vi "LabvolutionSubmoduleCheck_AddSubmoduleDialog.vi"(8 "error in (no error)":errorcluster, 11 "Project Dir":path) -> (0 "error out":errorcluster)   [LabVIEW 2018]
panel:
  in  "Select submodule parent folder":string(combo)
  in  "Cancel":bool
  in  "Add submodule":bool
  in  "Repository URL":string
  # "C:\\Users\\GregPayne\\Documents\\grp\\tmp\\submodule-demo"
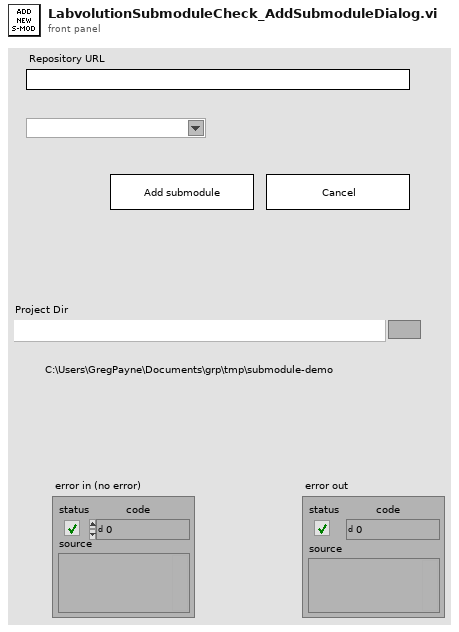
[diagram p1: front panel]
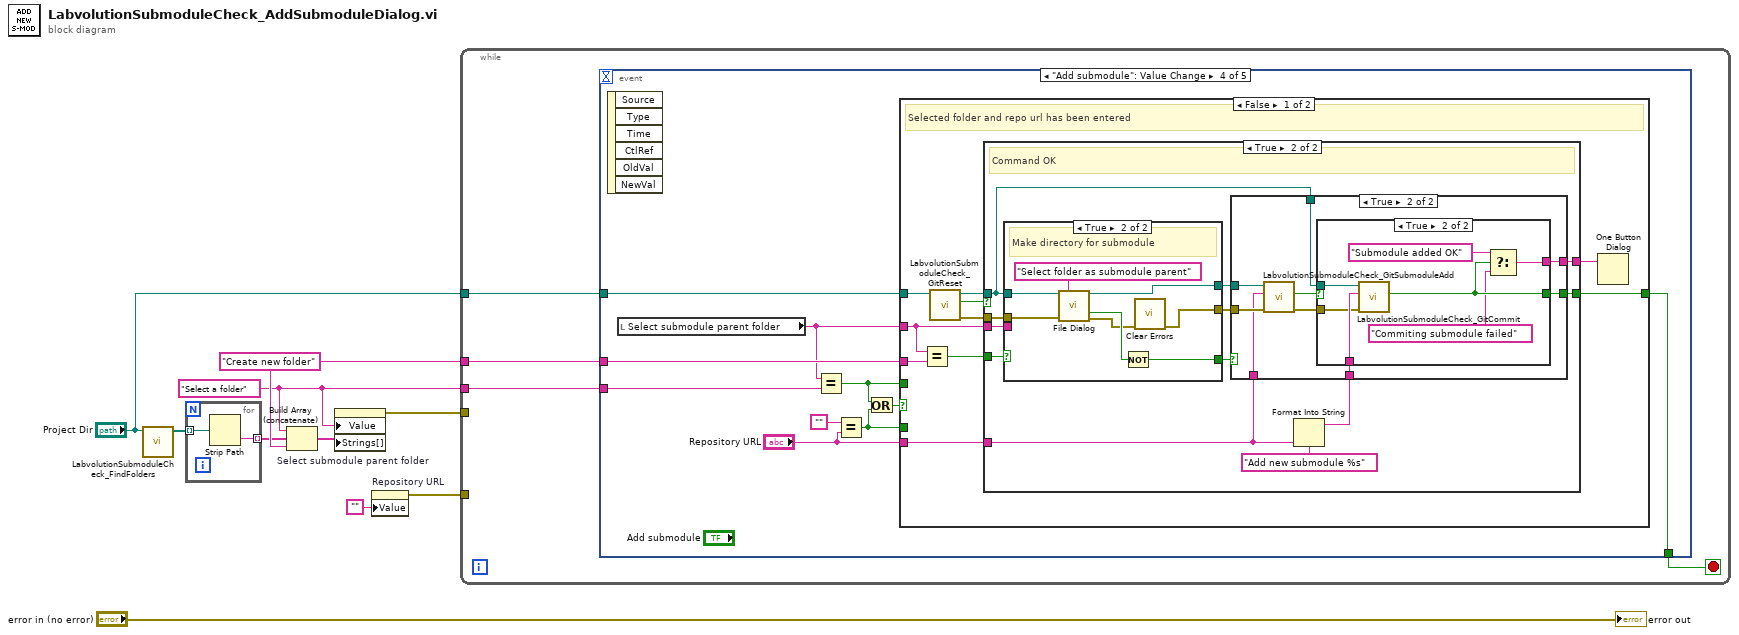
[diagram p0: block diagram]
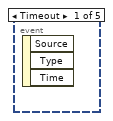
[diagram p2: hidden frame]
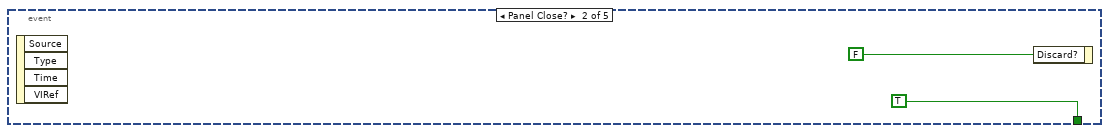
[diagram p3: hidden frame]
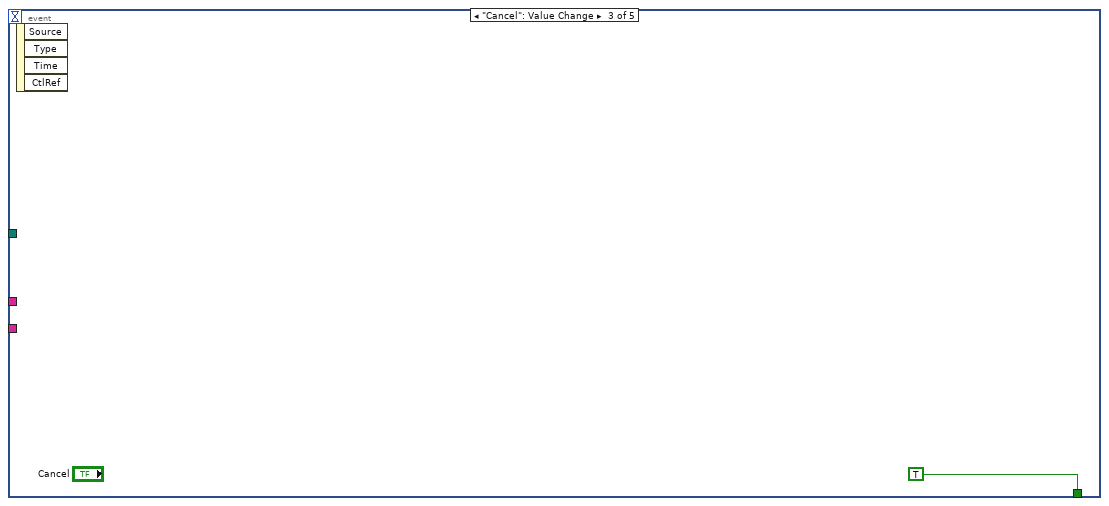
[diagram p4: hidden frame]
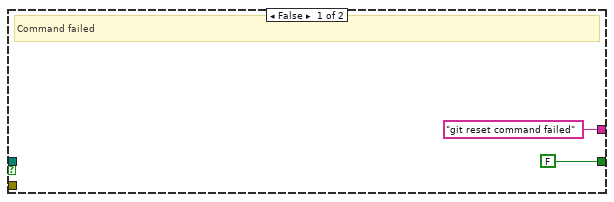
[diagram p5: hidden frame]
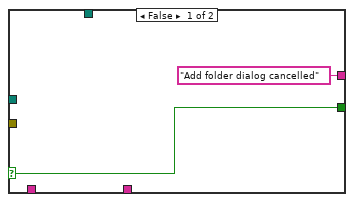
[diagram p6: hidden frame]
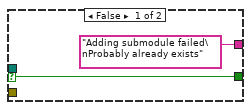
[diagram p7: hidden frame]
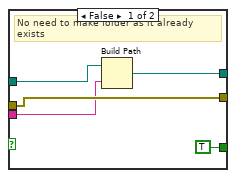
[diagram p8: hidden frame]
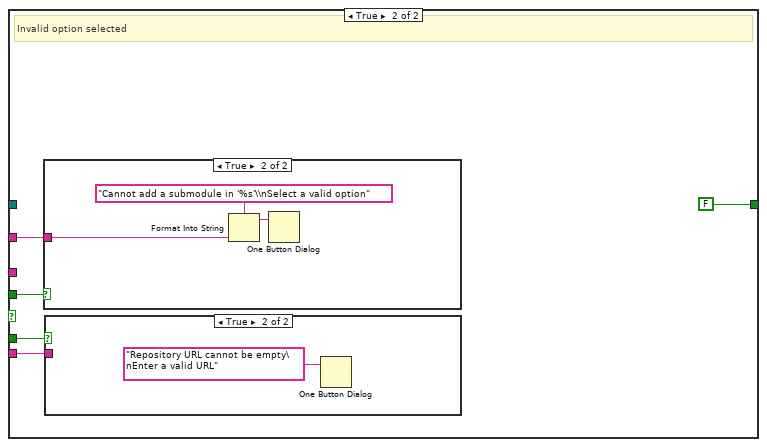
[diagram p9: hidden frame]
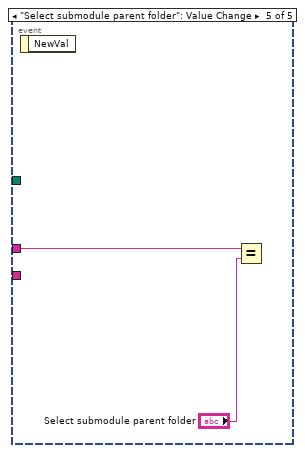
[diagram p12: hidden frame]
diagram:
  w6 = "Select a folder"
  w7 = "Create new folder"
  n1 = call "LabvolutionSubmoduleCheck_FindFolders.vi"("Project Dir"="Project Dir") -> ("Folders"=w1:path[])  [unwired: 10 in]
  n2 = for {
    tunnel: w1 -> [w11] mode=indexing
    tunnel: [w12] -> w5 mode=indexing
    n3 = Strip Path(path=w11) -> (name=w12:string)  [unwired: 1 out]
  }
  n4 = Build Array (concatenate)(w6, w5, w7) -> (w9:string[])
  n5 = property on="Select submodule parent folder" class="CmbBox"("Value"=w6, "Strings[]"=w9) -> (error out=w8:errorcluster)  [unwired: 2 in, 1 out]
  n6 = property on="Repository URL" class="Str"("Value"="") -> (error out=w3:errorcluster)  [unwired: 2 in, 1 out]
  n7 = while {
    tunnel: w8 -> [_]
    tunnel: w7 -> [w15]
    tunnel: w6 -> [w14]
    tunnel: "Project Dir" -> [w13]
    tunnel: w3 -> [_]
    stop <- w16 stop-if-true
    n8 = event shown="[3] \"Add submodule\": Value Change" {
      selector: _ -> [_ _ _ _ _]
      dyn-events: _ -> [_ _ _ _ _]
      timeout: _ -> [_ _ _ _ _]
      tunnel: [_ TRUE TRUE w26 _] -> w16
      tunnel: w15 -> [_ _ _ w29 w97]
      tunnel: w14 -> [_ _ _ w28 _]
      tunnel: w13 -> [_ _ _ w25 _]
      event Timeout {
        n9 = event-data() -> ()  [unwired: 1 in, 3 out]
      }
      event Panel Close? {
        n10 = event-data() -> ()  [unwired: 1 in, 4 out]
        n11 = event-data("Discard?"=FALSE) -> ()  [unwired: 1 in, 1 out]
      }
      event "Cancel": Value Change {
        n12 = event-data() -> ()  [unwired: 1 in, 4 out]
      }
      event "Add submodule": Value Change {
        n13 = event-data() -> ()  [unwired: 1 in, 6 out]
        n14 = local read "Select submodule parent folder"() -> (w27:string)
        n15 = Equal?(x=w27, y=w28) -> (x = y?=w21:bool)
        n16 = Equal?(x="", y="Repository URL") -> (x = y?=w20:bool)
        n17 = Or(x=w21, y=w20) -> (x .or. y?=w24:bool)
        n18 = case shown="False" w24 {
          tunnel: w29 -> [w39 _]
          tunnel: w27 -> [w35 w91]
          tunnel: [w37 FALSE] -> w26
          tunnel: w25 -> [w34 _]
          tunnel: "Repository URL" -> [w36 w87]
          tunnel: w21 -> [_ w89]
          tunnel: w20 -> [_ w88]
          frame False {
            # "Selected folder and repo url has been entered"
            n19 = Equal?(x=w35, y=w39) -> (x = y?=w38:bool)
            n20 = call "LabvolutionSubmoduleCheck_GitReset.vi"("Working Dir in"=w34) -> ("error out"=w33:errorcluster, "Command OK"=w32:bool, "Working Dir out"=w31:path)  [unwired: 8 in]
            n21 = case shown="True" w32 {
              tunnel: w38 -> [_ w53]
              tunnel: [FALSE w45] -> w37
              tunnel: w36 -> [_ w43]
              tunnel: w35 -> [_ w49]
              tunnel: w33 -> [_ w48]
              tunnel: w31 -> [_ w47]
              tunnel: ["git reset command failed" ("message") w42] -> w30
              frame False {
                # "Command failed"
              }
              frame True {
                # "Command OK"
                n22 = case shown="True" w53 {
                  tunnel: w47 -> [w75 w85]
                  tunnel: [TRUE w83] -> w44
                  tunnel: [w76 w82] -> w51
                  tunnel: [w77 w80] -> w52
                  tunnel: w48 -> [w77 w79]
                  tunnel: w49 -> [w74 _]
                  frame False {
                    # "No need to make folder as it already exists"
                    n23 = Build Path(base path=w75, name or relative path=w74) -> (appended path=w76:path)
                  }
                  frame True {
                    # "Make directory for submodule"
                    n24 = call "File Dialog"("start path"=w85, "prompt"="Select folder as submodule parent", "error in"=w79) -> ("selected path"=w82:path, "cancelled"=w84:bool, "error out"=w81:errorcluster)  [unwired: 9 in, 1 out]
                    n25 = Not(x=w84) -> (.not. x?=w83:bool)
                    n26 = call <vilib>:"Clear Errors.vi"("error in (no error)"=w81) -> ("error out"=w80:errorcluster)  [unwired: 5 in, 1 out]
                  }
                }
                n27 = Format Into String(format string="Add new submodule %s", w43) -> (resulting string=w46:string)  [unwired: 2 in, 1 out]
                n28 = case shown="True" w44 {
                  selector: w44 -> [w55 _]
                  tunnel: w43 -> [_ w58]
                  tunnel: w52 -> [_ w61]
                  tunnel: w51 -> [_ w60]
                  tunnel: w47 -> [_ w64]
                  tunnel: w46 -> [_ w63]
                  tunnel: [w55 w62] -> w45
                  tunnel: ["Add folder dialog cancelled" w56] -> w42
                  frame False {
                  }
                  frame True {
                    n29 = call "LabvolutionSubmoduleCheck_GitSubmoduleAdd.vi"("error in (no error)"=w61, "Repository URL"=w58, "Folder in"=w60) -> ("error out"=w59:errorcluster, "Command OK"=w57:bool)  [unwired: 6 in, 1 out]
                    n30 = case shown="True" w57 {
                      selector: w57 -> [w66 _]
                      tunnel: w64 -> [_ w73]
                      tunnel: w63 -> [_ w72]
                      tunnel: [w66 w70] -> w62
                      tunnel: w59 -> [_ w71]
                      tunnel: ["Adding submodule failed\nProbably already exists" ("format string") w69] -> w56
                      frame False {
                      }
                      frame True {
                        n31 = call "LabvolutionSubmoduleCheck_GitCommit.vi"("error in (no error)"=w71, "Message"=w72, "Working Dir in"=w73) -> ("Command OK"=w70:bool)  [unwired: 6 in, 2 out]
                        n32 = Select(t="Submodule added OK", s=w70, f="Commiting submodule failed" ("format string")) -> (s? t:f=w69:string)
                      }
                    }
                  }
                }
              }
            }
            n33 = One Button Dialog(message=w30) -> ()  [unwired: 1 in, 1 out]
          }
          frame True {
            # "Invalid option selected"
            n34 = case shown="True" w89 {
              tunnel: w91 -> [_ w94]
              frame False {
              }
              frame True {
                n35 = Format Into String(format string="Cannot add a submodule in '%s'\\nSelect a valid option" ("message"), w94) -> (resulting string=w93:string)  [unwired: 2 in, 1 out]
                n36 = One Button Dialog(message=w93) -> ()  [unwired: 1 in, 1 out]
              }
            }
            n37 = case shown="True" w88 {
              tunnel: w87 -> [_ _]
              frame False {
              }
              frame True {
                n38 = One Button Dialog(message="Repository URL cannot be empty\nEnter a valid URL") -> ()  [unwired: 1 in, 1 out]
              }
            }
          }
        }
      }
      event "Select submodule parent folder": Value Change {
        n39 = event-data() -> ()  [unwired: 1 in, 1 out]
        n40 = Equal?(x=w97, y="Select submodule parent folder") -> ()  [unwired: 1 out]
      }
    }
  }
  "error out" <- "error in (no error)"
